vi "qREC TRG.vi"(0 "System no.":i32=1 min=1 max=4 step=1, 2 "RecorderIDs to query":string[](array[string]), 5 "error in":errorcluster) -> (14 "List of Recorder Trigger Configurations":T1[](array[typedef]), 19 "error out":errorcluster)   [LabVIEW 2020]
doc: "REC? TRG (Get Data Recorder Trigger Information)\n\nDescription\nQueries the trigger configuration for the data recorders of the controller.\n\nFormat\nREC? TRG[ <RecorderID>]\n\nArguments\nREC? TRG without arguments queries all data recorders of the controller.\n<RecorderID>\nData recorder, whose configuration is to be queried; to be specified as alias (p. 94) \nThe available data recorders can be queried with USG? SYS (p. 80). \nPossible values: REC_1 to RECn, where n = number of data recorders in the controller\n\nResponse\n{<RecorderID>\"=\"<RecorderTrigger> <TriggerOption1> <TriggerOption2> LF}\nSee REC TRG (p. 40) for further details.\n\nExample\n>>rec? trg\n<<REC_1=MOV AXIS_1 1 \n<<REC_2=NOW - -\n>>rec? trg rec_1\n<<REC_1=MOV AXIS_1 1\n\nNotes\nFor further details, see \"Data Recorder - GCS 3.0\" (p. 107). \n\nUser command level\nUSR"
uses:
  RecorderTriggerConfiguration.ctl
panel:
  # "REC? TRG (Get Data Recorder Trigger Information)\n\nQueries the trigger configuration for the data recorders of the controller."
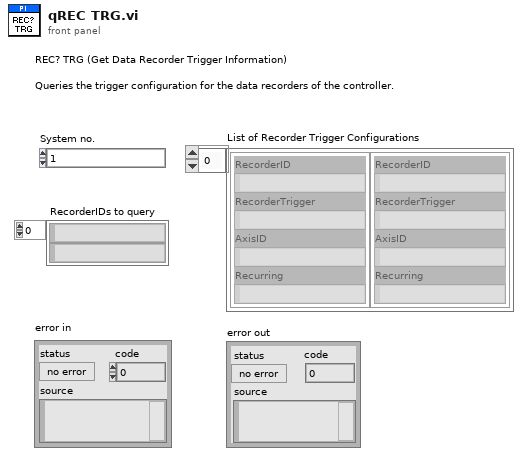
[diagram p1: front panel]
types:
  T1 = typedef "RecorderTriggerConfiguration.ctl" = cluster{"RecorderID":string, "RecorderTrigger":string, "AxisID":string, "Recurring":string}
  T2 = typedef "Syntax.ctl" = enum16{"GCS 1.0", "GCS 2.0", "GCS 3.0"}
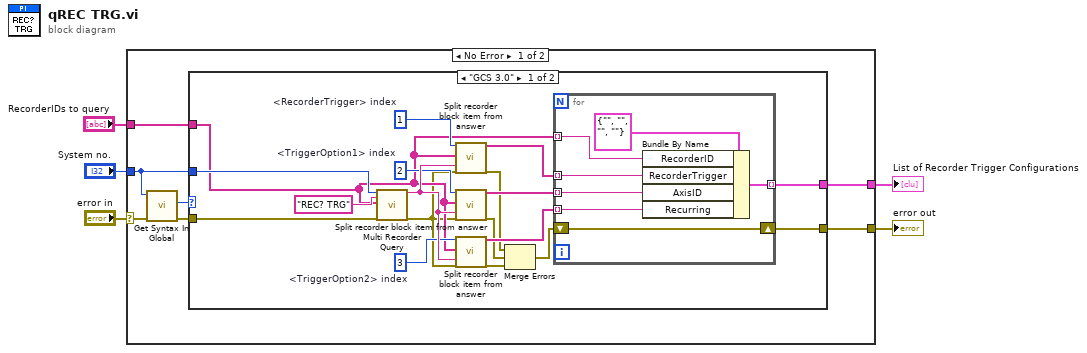
[diagram p0: block diagram]
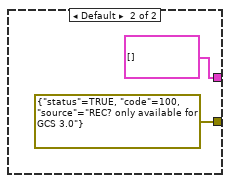
[diagram p2: hidden frame]
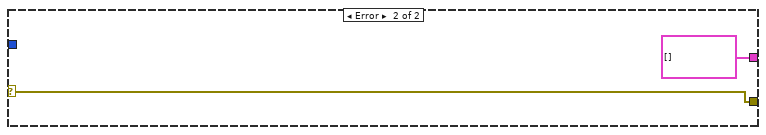
[diagram p3: hidden frame]
diagram:
  n1 = case shown="No Error" "error in" {
    selector: "error in" -> [w12 w41]
    tunnel: [w9 w41] -> w4
    tunnel: "RecorderIDs to query" -> [w7 _]
    tunnel: "System no." -> [w6 _]
    tunnel: [w8 T1[] [] ("List of Recorder Trigger Configurations")] -> w1
    frame No Error {
      n2 = call "Get Syntax In Global.vi"("error in"=w12, "System no."=w6) -> ("error out"=w10:errorcluster, "Syntax"=w11:T2)  [unwired: 8 in]
      n3 = case shown="\"GCS 3.0\"" w11 {
        tunnel: w10 -> [w28 _]
        tunnel: [w23 errorcluster {"status"=TRUE, "code"=100, "source"="REC? only available for GCS 3.0"} ("error out")] -> w9
        tunnel: [w19 T1[] [] ("List of Recorder Trigger Configurations")] -> w8
        tunnel: w7 -> [w18 _]
        tunnel: w6 -> [w30 _]
        frame "GCS 3.0" {
          w24 = 3  # <TriggerOption2> index
          w25 = 2  # <TriggerOption1> index
          w27 = 1  # <RecorderTrigger> index
          n4 = call "Multi Recorder Query.vi"("System no."=w30, "Recorder Command"="REC? TRG" ("format string"), "RecorderIDs to query"=w18, "error in"=w28) -> ("Answer"=w26:string, "error out"=w13:errorcluster)  [unwired: 14 in]
          n5 = call "Split recorder block item from answer.vi"("Slice block item"=w27, "RecorderIDs to query"=w18, "Input string"=w26, "error in"=w13) -> ("Sliced text segments"=w22:string[], "error out"=w17:errorcluster)  [unwired: 14 in]
          n6 = call "Split recorder block item from answer.vi"("Slice block item"=w25, "RecorderIDs to query"=w18, "Input string"=w26, "error in"=w13) -> ("Sliced text segments"=w21:string[], "error out"=w16:errorcluster)  [unwired: 14 in]
          n7 = call "Split recorder block item from answer.vi"("Slice block item"=w24, "RecorderIDs to query"=w18, "Input string"=w26, "error in"=w13) -> ("Sliced text segments"=w20:string[], "error out"=w15:errorcluster)  [unwired: 14 in]
          n8 = Merge Errors(w17, w16, w15) -> (w14:errorcluster)
          n9 = for {
            shift-right: [w37] -> w23
            shift-left: w14 -> [w37]
            tunnel: w22 -> [w33] mode=indexing
            tunnel: w21 -> [w32] mode=indexing
            tunnel: w20 -> [w34] mode=indexing
            tunnel: [w36] -> w19 mode=indexing
            tunnel: w18 -> [w35] mode=indexing
            n10 = Bundle By Name(cluster=T1 {"RecorderID"="", "RecorderTrigger"="", "AxisID"="", "Recurring"=""} ("RecorderTriggerConfiguration"), "RecorderID"=w35, "RecorderTrigger"=w33, "AxisID"=w32, "Recurring"=w34) -> (w36:T1)
          }
        }
        frame Default {
        }
      }
    }
    frame Error {
    }
  }
  "error out" <- w4
  "List of Recorder Trigger Configurations" <- w1
